vi "Cont Acq&Graph Voltage-Int Clk Make Waveform from 2D LV2012 NIVerified.vi"() -> ()   [LabVIEW 2020]
doc: "I. Description:\nThis example demonstrates how to acquire a continuous amount of data (Waveform) using the DAQ device's internal clock.\n\nII. Instructions for Running:\n1. Create an analog input voltage channel.\n2. Set the rate for the sample clock. Additionally, define the sample mode to be continuous.\n3. Call the Start VI to start the acquisition.\n4. Read the waveform data in a loop until the user hits the stop button or an error occurs.\nNote: This example reads data from one or more channels and returns an array of data. Use the Index Array function to access an individual channel of data.\n5. Call the Clear Task VI to clear the Task.\n6. Use the popup dialog box to display an error if any.\n\nIV. I/O Connections Overview:\nMake sure your signal input terminal matches the Physical Channel I/O Control. For further connection information, refer to your hardware reference manual."
uses:
  <vilib>/Utility/error.llb/DialogType.ctl
  <vilib>/DAQmx/read.llb/DAQmx Read (Analog 2D DBL NChan NSamp).vi
  <vilib>/DAQmx/create/channels.llb/DAQmx Create Channel (AI-Voltage-Basic).vi
  <vilib>/DAQmx/configure/timing.llb/DAQmx Timing (Sample Clock).vi
  <vilib>/DAQmx/miscellaneous.llb/DAQmx Fill In Error Info.vi
panel:
  out "Measurement":waveform(dbl)[](graph)
  in  "Samples to Read":i32=1000
  in  "Physical Channel":tag="Dev1/ai0"
  in  "Minimum Value":dbl=-10.0 format="%0.2f"
  in  "Maximum Value":dbl=10.0 format="%0.2f"
  in  "stop":bool
  in  "Sample Rate":dbl=10000.0 caption="Sample Rate (Hz)" format="%0.2f"
  # "Overview\n  This example converts the datatype of a 2D array of raw data into a 1D array of waveforms for use with 3rd party devices. \nRequirements\nSoftware\n   LabVIEW 2012 or compatible\n   NI-DAQmx 9.5.5 or compatible \nHardware\n   NI Multifuntion DAQ Device\nInstructions\n  1.Configure the parameter for the right channel and device\n  2.Connect your hardware appropriately\n  3.Run the VI"
  # "For instructions, select Help>>Show Context Help"
  # "Channel Parameters"
  # "Timing Parameters"
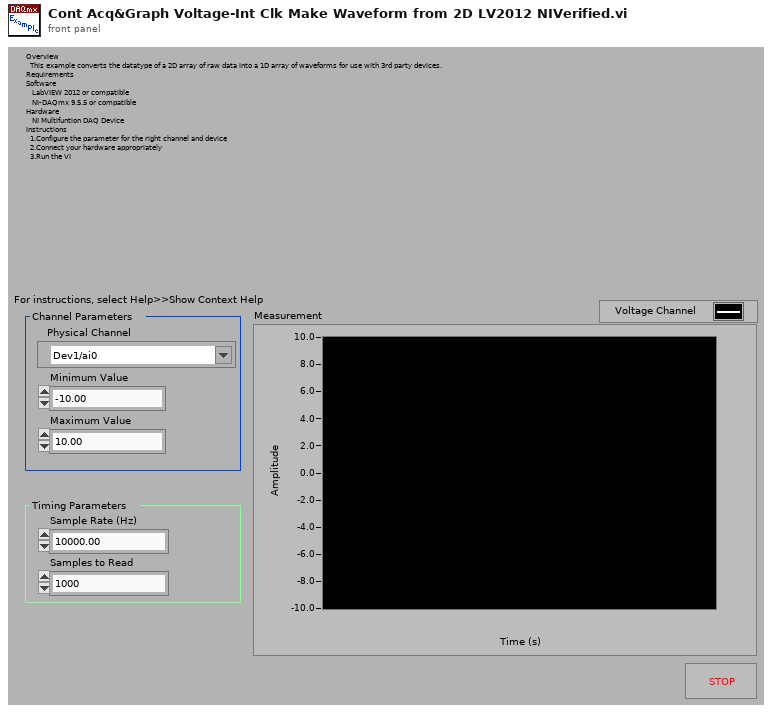
[diagram p1: front panel]
types:
  T1 = typedef "DialogType.ctl" = u16
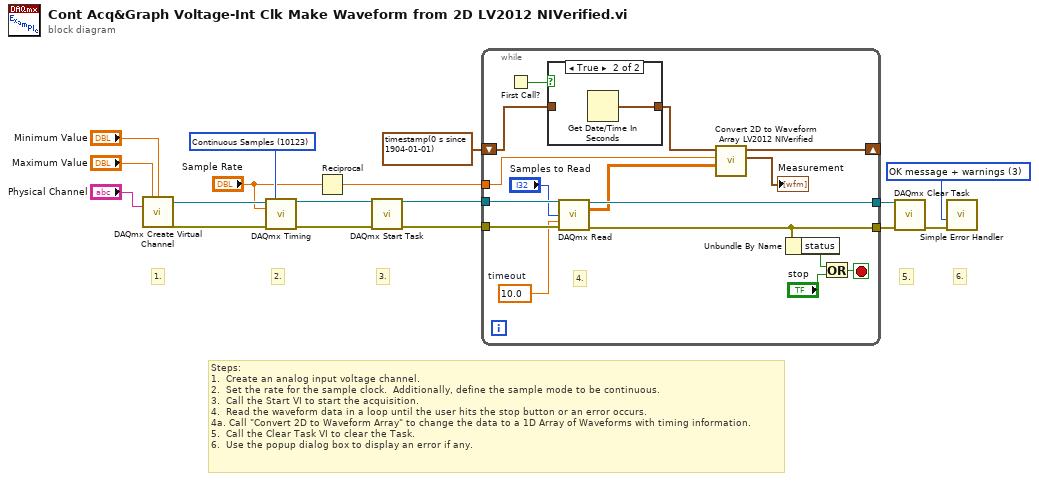
[diagram p0: block diagram]
diagram:
  w4 = T1 3 items=["no dialog", "OK message", "continue or stop message", "OK message + warnings", "continue/stop + warnings"] ("type of dialog (OK msg:1)")
  w8 = 10123 items=["Finite Samples"=10178, "Continuous Samples"=10123] ("sample mode")
  # "6."
  # "5."
  # "Steps: \n1.  Create an analog input voltage channel.\n2.  Set the rate for the sample clock.  Additionally, define the sample mode to be continuous.\n3.  Call the Start VI to start the acquisition.\n4.  Read the waveform data in a loop until the user hits the stop button or an error occurs.\n4a. Call \"Convert 2D to Waveform Array\" to change the data to a 1D Array of Waveforms with timing information.\n5.  Call the Clear Task VI to clear the Task.\n6.  Use the popup dialog box to display an error if any."
  # "3."
  # "2."
  # "1."
  n1 = call-poly <vilib>:"DAQmx Create Virtual Channel.vi"("maximum value"="Maximum Value", "minimum value"="Minimum Value", "physical channels"="Physical Channel") -> ("task out"=w12:refnum<k21>, "error out"=w15:errorcluster)  [unwired: 11 in]
  n2 = call-poly <vilib>:"DAQmx Timing.vi"("task/channels in"=w12, "sample mode"=w8, "rate"="Sample Rate", "error in"=w15) -> ("task out"=w7:refnum<k21>, "error out"=w6:errorcluster)  [unwired: 10 in]
  n3 = Reciprocal(x="Sample Rate") -> (1/x=w2:dbl)
  n4 = call <vilib>:"DAQmx Start Task.vi"("task/channels in"=w7, "error in"=w6) -> ("task out"=w11:refnum<k21>, "error out"=w14:errorcluster)  [unwired: 12 in]
  n5 = while {
    tunnel: w14 -> [w33]
    tunnel: w11 -> [w32]
    tunnel: [w31] -> w10
    tunnel: [w30] -> w5
    shift-right: [w22] -> _
    shift-left: timestamp(0 s since 1904-01-01) ("New t0") -> [w19]
    tunnel: w2 -> [w21]
    stop <- w28 stop-if-true
    w26 = 10.0  # timeout
    # "4."
    n6 = First Call?() -> (First Call?: T/F=w23:bool)
    n7 = case shown="True" w23 {
      tunnel: [w34 w35] -> w20
      tunnel: w19 -> [w34 _]
      frame False {
      }
      frame True {
        n8 = Get Date/Time In Seconds() -> (seconds since 1Jan1904=w35:timestamp)
      }
    }
    n9 = call-poly <vilib>:"DAQmx Read.vi"("task/channels in"=w32, "number of samples per channel"="Samples to Read", "timeout"=w26, "error in"=w33) -> ("task out"=w31:refnum<k21>, "data"=w24:dbl[][], "error out"=w30:errorcluster)  [unwired: 9 in]
    n10 = call "Convert 2D to Waveform Array LV2012 NIVerified.vi"("Data"=w24, "dt"=w21, "t0"=w20) -> ("Waveform Array Out"=→"Measurement":waveform(dbl)[], "New t0"=w22:timestamp)  [unwired: 7 in]
    n11 = Unbundle By Name(w30) -> ("status"=w29:bool)
    n12 = Or(x=w29, y="stop") -> (x .or. y?=w28:bool)
  }
  n13 = call <vilib>:"DAQmx Clear Task.vi"("task in"=w10, "error in"=w5) -> ("error out"=w13:errorcluster)  [unwired: 13 in]
  n14 = call <vilib>:"Simple Error Handler.vi"("type of dialog (OK msg:1)"=w4, "error in (no error)"=w13) -> ()  [unwired: 3 in, 5 out]
